vi "View Holder.vi"(8 "error in (no error)":errorcluster, 10 "Context":refnum<class "Debug Process.lvclass">, 11 "Debug View in":refnum<class "Debug View.lvclass">) -> (0 "error out":errorcluster, 3 "Debug View out":refnum<class "Debug View.lvclass">)   [LabVIEW 2020, in "Debug View.lvclass"]
uses:
  Debug View.lvclass
  Process/Debug Process.lvclass
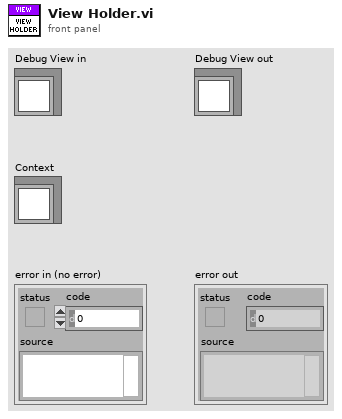
[diagram p1: front panel]
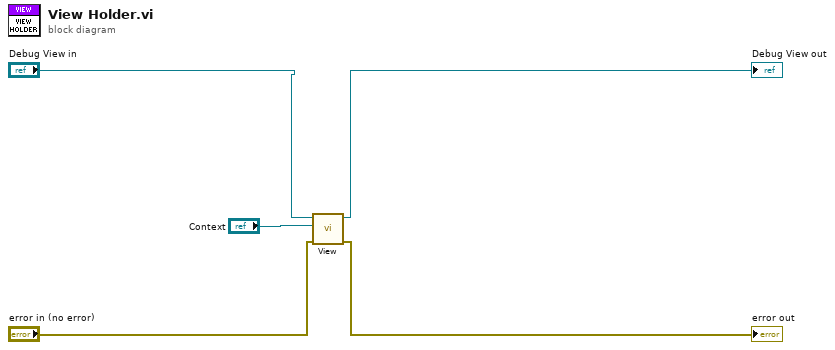
[diagram p0: block diagram]
diagram:
  n1 = call-dynamic "View.vi"("error in (no error)"="error in (no error)", "Context"="Context", "Debug View in"="Debug View in") -> ("error out"=→"error out":errorcluster, "Debug View out"=→"Debug View out":refnum<class "Debug View.lvclass">)  [unwired: 7 in]
